vi "Command Handler Global.vi"() -> ()   [LabVIEW 2015, in "Command Handler.lvlib"]
uses:
  Command Handler.lvlib
panel:
  out "Command Handling Disabled":bool
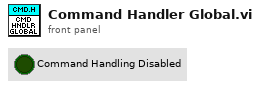
[diagram p1: front panel]
diagram:
